vi "connectPubDataSubscribe.vi"(8 "error in (no error)":errorcluster, 11 "MiddlewareSVThisComponent in":refnum<class "MiddlewareSVThisComponent.lvclass">) -> (0 "error out":errorcluster, 3 "MiddlewareSVThisComponent out":refnum<class "MiddlewareSVThisComponent.lvclass">)   [LabVIEW 2015, in "MiddlewareSVThisComponent.lvclass"]
uses:
  MiddlewareSVThisComponent.lvclass
  ComponentTemplateCore/ComponentModel/ComponentModel/Typedefs/CommunicationConfig.ctl
  ComponentTemplateCore/ComponentModel/ComponentModel/Typedefs/SVProcessConfig.ctl
  ComponentTemplateCore/ComponentModel/ComponentModelDT/ConfigurationFileReaderDT/ConfigurationFileReaderDT.lvclass
  ComponentTemplateCore/ComponentModel/ComponentModelRT/ConfigurationFileReaderRT/ConfigurationFileReaderRT.lvclass
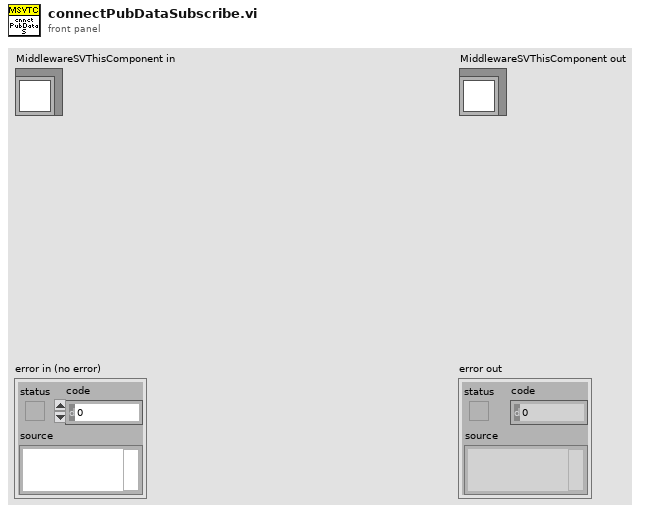
[diagram p1: front panel]
types:
  T1 = typedef "SVProcessConfig.ctl" = cluster{"subDataProcessPrototype":string, "pubDataProcessPrototype":string, "commandProcessPrototype":string, "commandSVName":string}
  T2 = typedef "CommunicationConfig.ctl" = cluster{"hostComputerAddress":string, "ComponentAcronym":string, "InstanceIdentifier":i32}
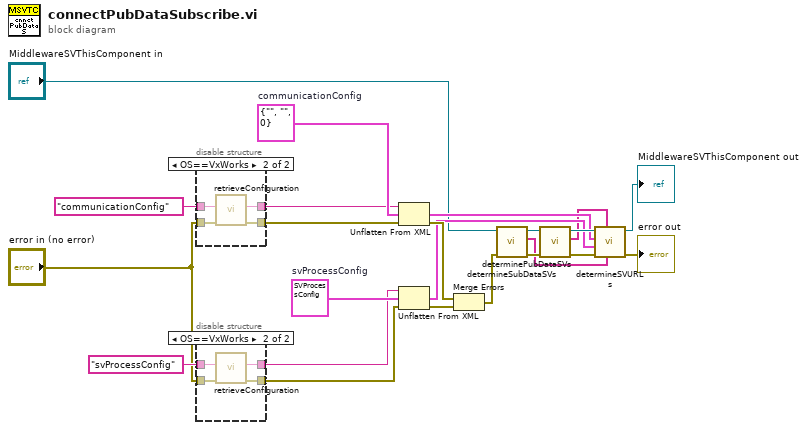
[diagram p0: block diagram]
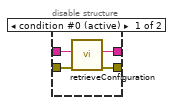
[diagram p2: hidden frame]
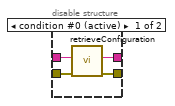
[diagram p3: hidden frame]
diagram:
  w22 = T1 {"subDataProcessPrototype"="SubDataSV", "pubDataProcessPrototype"="PubDataSV", "commandProcessPrototype"="CommandSV", "commandSVName"="Command"}  # svProcessConfig
  w23 = T2 {"hostComputerAddress"="", "ComponentAcronym"="", "InstanceIdentifier"=0}  # communicationConfig
  n1 = disable-structure shown="OS==VxWorks" {
    disable-tunnel: "communicationConfig" ("dataName") -> [w27 w31]
    disable-tunnel: [w26 w29] -> w15
    disable-tunnel: [w25 w28] -> w14
    disable-tunnel: "error in (no error)" -> [w24 w30]
    frame condition #0 (active) {
      n2 = call "retrieveConfiguration.vi"("error in (no error)"=w24, "dataName"=w27) -> ("error out"=w25:errorcluster, "dataValueFromFile"=w26:string)  [unwired: 7 in, 1 out]
    }
    frame condition #1 {
      n3 = call "retrieveConfiguration.vi"("error in (no error)"=w30, "dataName"=w31) -> ("error out"=w28:errorcluster, "dataValueFromFile"=w29:string)  [unwired: 7 in, 1 out]
    }
  }
  n4 = disable-structure shown="OS==VxWorks" {
    disable-tunnel: "svProcessConfig" ("dataName") -> [w35 w39]
    disable-tunnel: [w34 w37] -> w12
    disable-tunnel: [w33 w36] -> w11
    disable-tunnel: "error in (no error)" -> [w32 w38]
    frame condition #0 (active) {
      n5 = call "retrieveConfiguration.vi"("error in (no error)"=w32, "dataName"=w35) -> ("error out"=w33:errorcluster, "dataValueFromFile"=w34:string)  [unwired: 7 in, 1 out]
    }
    frame condition #1 {
      n6 = call "retrieveConfiguration.vi"("error in (no error)"=w38, "dataName"=w39) -> ("error out"=w36:errorcluster, "dataValueFromFile"=w37:string)  [unwired: 7 in, 1 out]
    }
  }
  n7 = Unflatten From XML(xml string=w15, type=w23, error in (no error)=w14) -> (value=w17:T2, error out=w21:errorcluster)
  n8 = Unflatten From XML(xml string=w12, type=w22, error in (no error)=w11) -> (value=w16:T1, error out=w20:errorcluster)
  n9 = Merge Errors(w21, w20) -> (w5:errorcluster)
  n10 = call "determineSubDataSVs.vi"("error in (no error)"=w5, "MiddlewareSVThisComponent in"="MiddlewareSVThisComponent in") -> ("error out"=w3:errorcluster, "svNames"=w2:string[], "MiddlewareSVThisComponent out"=w4:refnum<class "MiddlewareSVThisComponent.lvclass">)  [unwired: 7 in]
  n11 = call "determinePubDataSVs.vi"("error in (no error)"=w3, "MiddlewareSVThisComponent in"=w4) -> ("error out"=w19:errorcluster, "svNames"=w1:string[], "MiddlewareSVThisComponent out"=w18:refnum<class "MiddlewareSVThisComponent.lvclass">)  [unwired: 7 in]
  n12 = call-dynamic "determineSVURLs.vi"("subDataSVNames"=w2, "pubDataSVNames"=w1, "error in (no error)"=w19, "svProcessConfig"=w16, "communicationConfig"=w17, "MiddlewareSV in"=w18) -> ("error out"=→"error out":errorcluster, "MiddlewareSV out"=→"MiddlewareSVThisComponent out":refnum<class "MiddlewareSVThisComponent.lvclass">)  [unwired: 4 in]
